vi "Control Mode Select Power Supply.vi"(8 "Control Mode Read":u16, 9 "Power Read":dbl, 10 "Voltage Read":dbl, 11 "Current Read":dbl) -> (1 "Power Write":dbl, 2 "Voltage Write":dbl, 3 "Current Write":dbl)   [LabVIEW 2023]
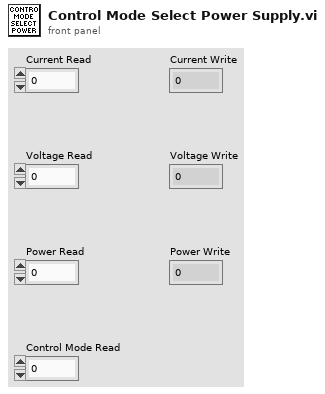
[diagram p1: front panel]
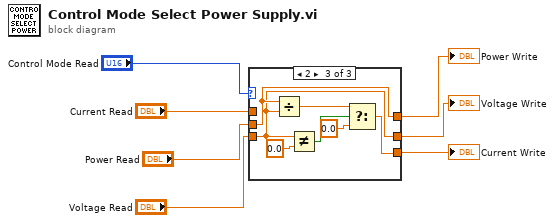
[diagram p0: block diagram]
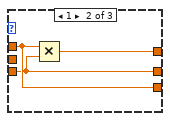
[diagram p3: hidden frame]
diagram:
  n1 = case shown="2" "Control Mode Read" {
    tunnel: "Current Read" -> [w10 w13 _]
    tunnel: [w10 w13 w14] -> w7
    tunnel: "Voltage Read" -> [w9 w12 w16]
    tunnel: [w9 w12 w16] -> w6
    tunnel: [w8 w11 w17] -> w5
    tunnel: "Power Read" -> [w8 _ w17]
    frame 0, Default {
    }
    frame 1 {
      n2 = Multiply(x=w13, y=w12) -> (x*y=w11:dbl)
    }
    frame 2 {
      n3 = Divide(x=w17, y=w16) -> (x/y=w18:dbl)
      n4 = Not Equal?(x=w16, y=0.0) -> (x != y?=w19:bool)
      n5 = Select(t=w18, s=w19, f=0.0) -> (s? t:f=w14:dbl)
    }
  }
  "Current Write" <- w7
  "Voltage Write" <- w6
  "Power Write" <- w5
